vi "Clean List of Properties Tree by Type.vi"(11 "Data Cluster in":T1) -> (0 "List of Tags":string[](array[string]), 3 "output cluster":T1)   [LabVIEW 2020, in "Control Property Tree.lvlib"]
uses:
  Control Property Tree.lvlib
  Module Data--cluster.ctl
  Ctrl Properties Map Data.ctl
  Property array.ctl
  Selected Ctrls - List of Controls.ctl
  Selected Ctrls - List of Properties.ctl
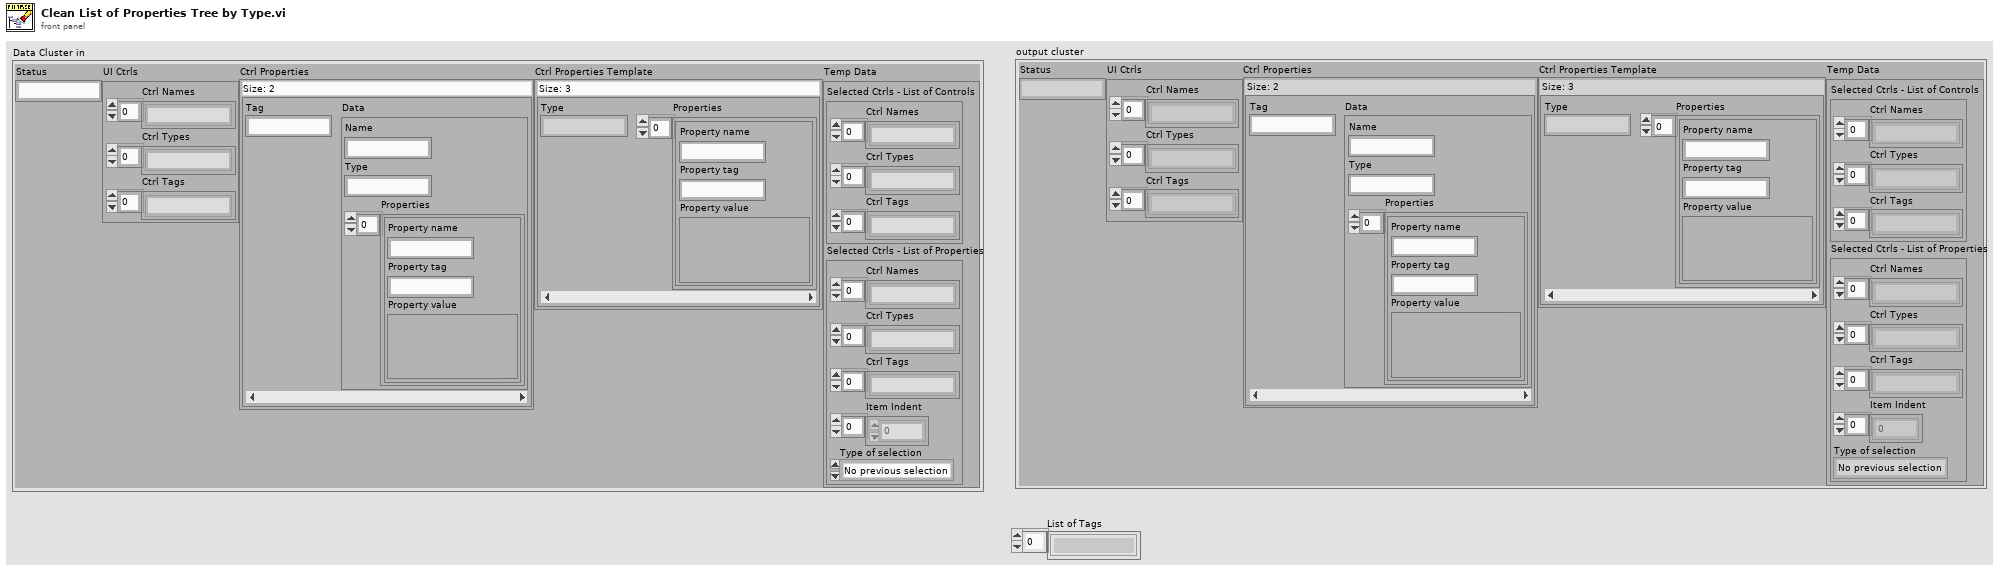
[diagram p1: front panel]
types:
  T1 = typedef "Control Property Tree.lvlib/Module Data--cluster.ctl" = cluster{"Status":string, "UI Ctrls":cluster{"Ctrl Names":string[], "Ctrl Types":string[], "Ctrl Tags":string[]}, "Ctrl Properties":map{string, T2}, "Ctrl Properties Template":map{string, T3}, "Temp Data":cluster{"Selected Ctrls - List of Controls":T4, "Selected Ctrls - List of Properties":T5}}
  T2 = typedef "Control Property Tree.lvlib/Ctrl Properties Map Data.ctl" = cluster{"Name":string, "Type":string, "Properties":T3}
  T3 = typedef "Control Property Tree.lvlib/Property array.ctl" = cluster{"Property name":string, "Property tag":string, "Property value":variant}[]
  T4 = typedef "Control Property Tree.lvlib/Selected Ctrls - List of Controls.ctl" = cluster{"Ctrl Names":string[], "Ctrl Types":string[], "Ctrl Tags":string[]}
  T5 = typedef "Control Property Tree.lvlib/Selected Ctrls - List of Properties.ctl" = cluster{"Ctrl Names":string[], "Ctrl Types":string[], "Ctrl Tags":string[], "Item Indent":i32[], "Type of selection":enum16{"No previous selection", "Control selected", "Property selected"}}
  T6 = enum16{"No previous selection", "Control selected", "Property selected"}
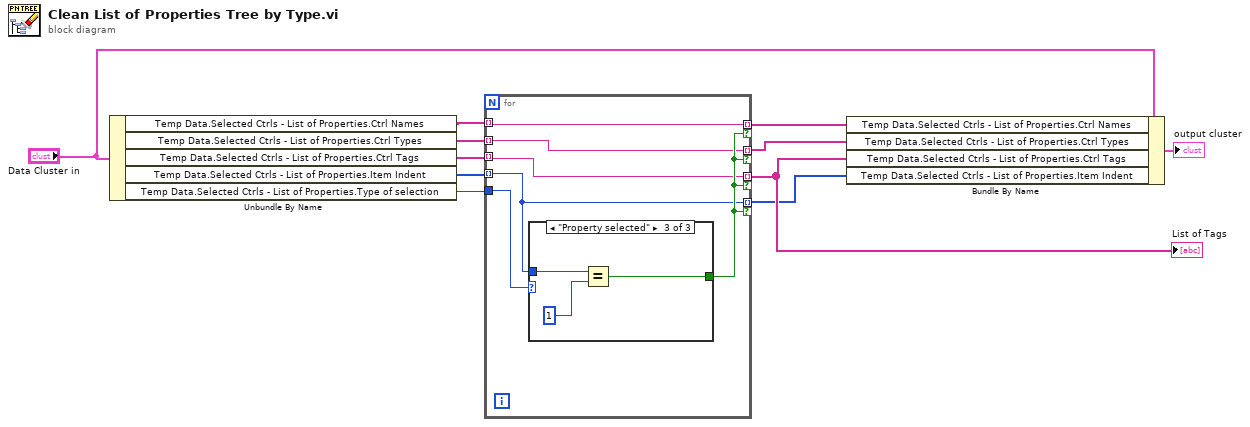
[diagram p0: block diagram]
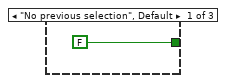
[diagram p2: hidden frame]
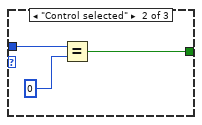
[diagram p3: hidden frame]
diagram:
  n1 = Unbundle By Name("Data Cluster in") -> ("Temp Data.Selected Ctrls - List of Properties.Ctrl Names"=w5:string[], "Temp Data.Selected Ctrls - List of Properties.Ctrl Types"=w4:string[], "Temp Data.Selected Ctrls - List of Properties.Ctrl Tags"=w3:string[], "Temp Data.Selected Ctrls - List of Properties.Item Indent"=w2:i32[], "Temp Data.Selected Ctrls - List of Properties.Type of selection"=w1:T6)
  n2 = for {
    tunnel: w4 -> [w14] mode=indexing
    tunnel: w5 -> [w15] mode=indexing
    tunnel: w3 -> [w13] mode=indexing
    tunnel: w2 -> [w12] mode=indexing
    tunnel: w1 -> [w17]
    tunnel: [w15] -> w11 mode=indexing if=w16
    tunnel: [w14] -> w10 mode=indexing if=w16
    tunnel: [w13] -> w9 mode=indexing if=w16
    tunnel: [w12] -> w8 mode=indexing if=w16
    n3 = case shown="\"Property selected\"" w17 {
      tunnel: w12 -> [_ w20 w23]
      tunnel: [FALSE w19 w22] -> w16
      frame "No previous selection", Default {
      }
      frame "Control selected" {
        n4 = Equal?(x=w20, y=0) -> (x = y?=w19:bool)
      }
      frame "Property selected" {
        n5 = Equal?(x=w23, y=1) -> (x = y?=w22:bool)
      }
    }
  }
  "List of Tags" <- w9
  n6 = Bundle By Name(cluster="Data Cluster in", "Temp Data.Selected Ctrls - List of Properties.Ctrl Names"=w11, "Temp Data.Selected Ctrls - List of Properties.Ctrl Types"=w10, "Temp Data.Selected Ctrls - List of Properties.Ctrl Tags"=w9, "Temp Data.Selected Ctrls - List of Properties.Item Indent"=w8) -> (→"output cluster":T1)
